vi "Nonlinear Calibration Test v4.vi"() -> ()   [LabVIEW 2009]
doc: "This example illustrates the use of a calibration grid to calibrate and correct an image for nonlinear distortion and accurate shape measurements.\n\nThis example loads the image of a calibration grid used to calibrate the system, learns the grid, then loads an image of parts acquired using the same setup. The example then corrects the image in two ways. The first method corrects the entire image and then measures the area of the coins. The second method corrects only the area of the coins and displays the difference in processing time."
uses:
  <vilib>/userDefined/High Color/IMAQdx.ctl
  <vilib>/vision/NI_Vision_Development_Module.lvlib
  <vilib>/vision/driver/NI_Vision_Acquisition_Software.lvlib
panel:
  in  "Camera Name":T1
  in  "Video Modes":i32(listbox)
  in  "stop":bool
  out "Image":T2(plugin-control)
  out "Buffer Number":u32
  out "Frame Rate":dbl(knob) scale=0.0..100.0 scale format="%.1f"
  in  "Red Range":cluster{"Lower value":i32, "Upper value":i32}={"Lower value"=240, "Upper value"=255}
  in  "Green Range":cluster{"Lower value":i32, "Upper value":i32}={"Lower value"=250, "Upper value"=255}
  in  "Blue Range":cluster{"Lower value":i32, "Upper value":i32}={"Lower value"=250, "Upper value"=255}
  in  "Color Mode":u16(ring) items=["RGB", "HSL", "HSV", "HSI"]
  out "Super Filter":T2(plugin-control)
  in  "File Path 2":path
  in  "File Path":path
  out "Bottom Image":T2(plugin-control) caption="Calibrated Measurements"
  out "Top Image":T2(plugin-control) caption="Corrected Image"
  # "This step takes measurements in two ways.  The first calculation corrects \nthe entire image, and then takes the measurements.  The second calculation only corrects the coins, and then takes the measurements."
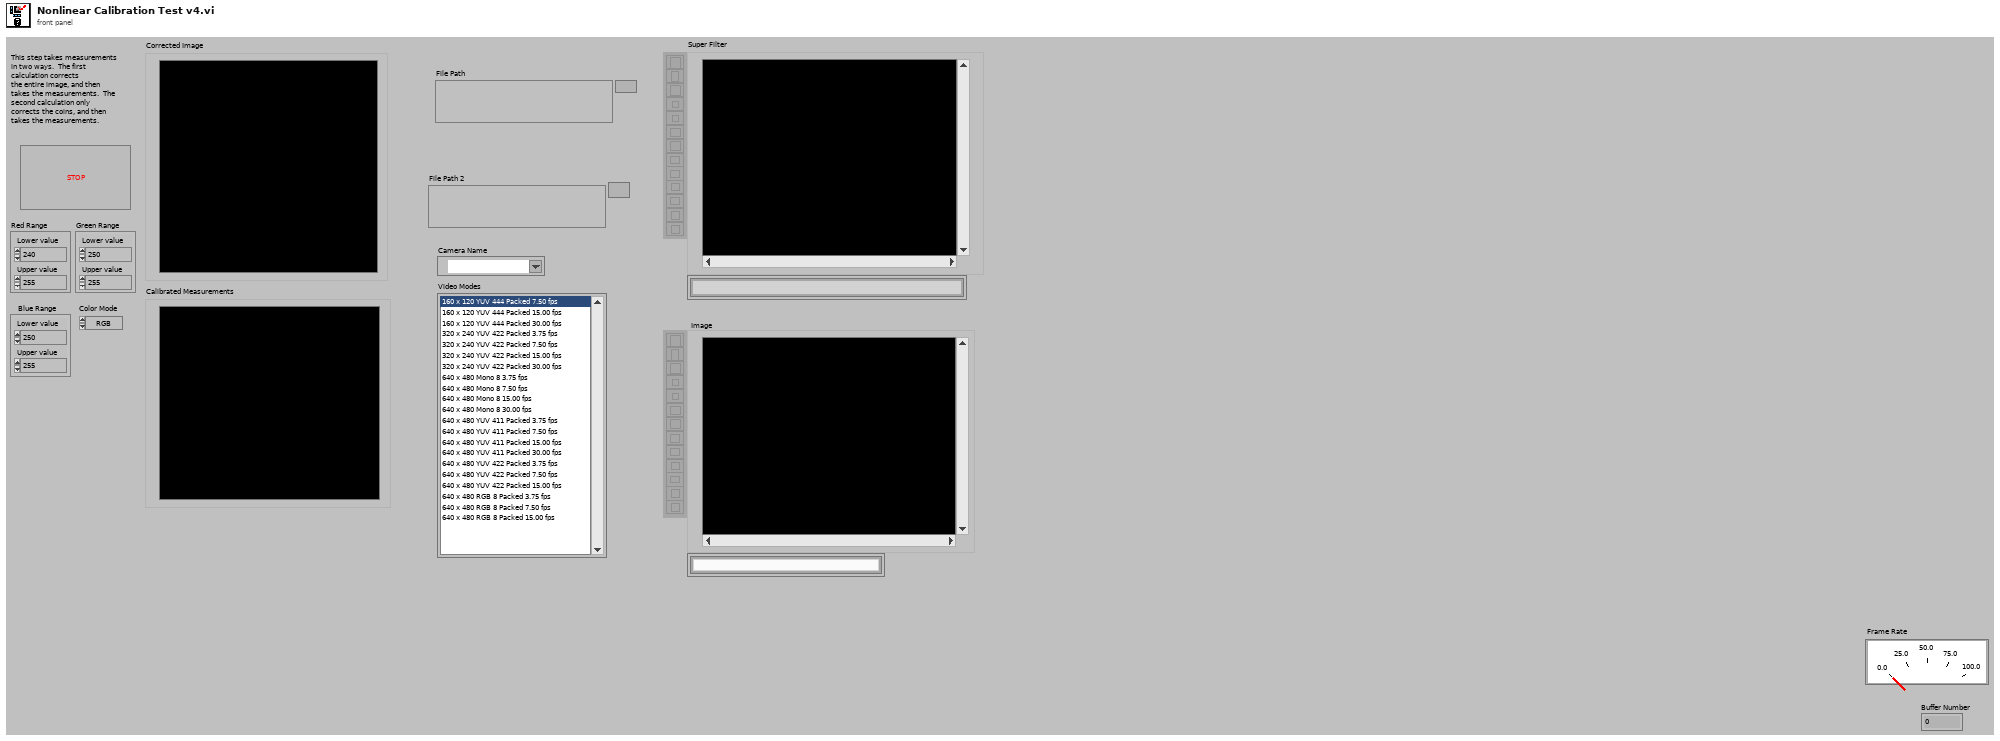
[diagram p1: front panel]
types:
  T1 = typedef "IMAQdx.ctl" = refnum<k21>
  T2 = typedef "IMAQ Image.ctl" = refnum<image>
  T3 = typedef "Image Type" = u32
  T4 = cluster{"X Step":sgl, "Y Step":sgl, "Unit":u32, "Threshold Range":cluster{"Lower value":sgl, "Upper value":sgl}}
  T5 = cluster{"Distortion":u32, "Corrected Image Scaling":u32, "Corrected Image Learn ROI":u32, "Learn Error Map?":bool, "Learn Correction Table?":bool}
  T6 = typedef "Particle Parameters" = i32
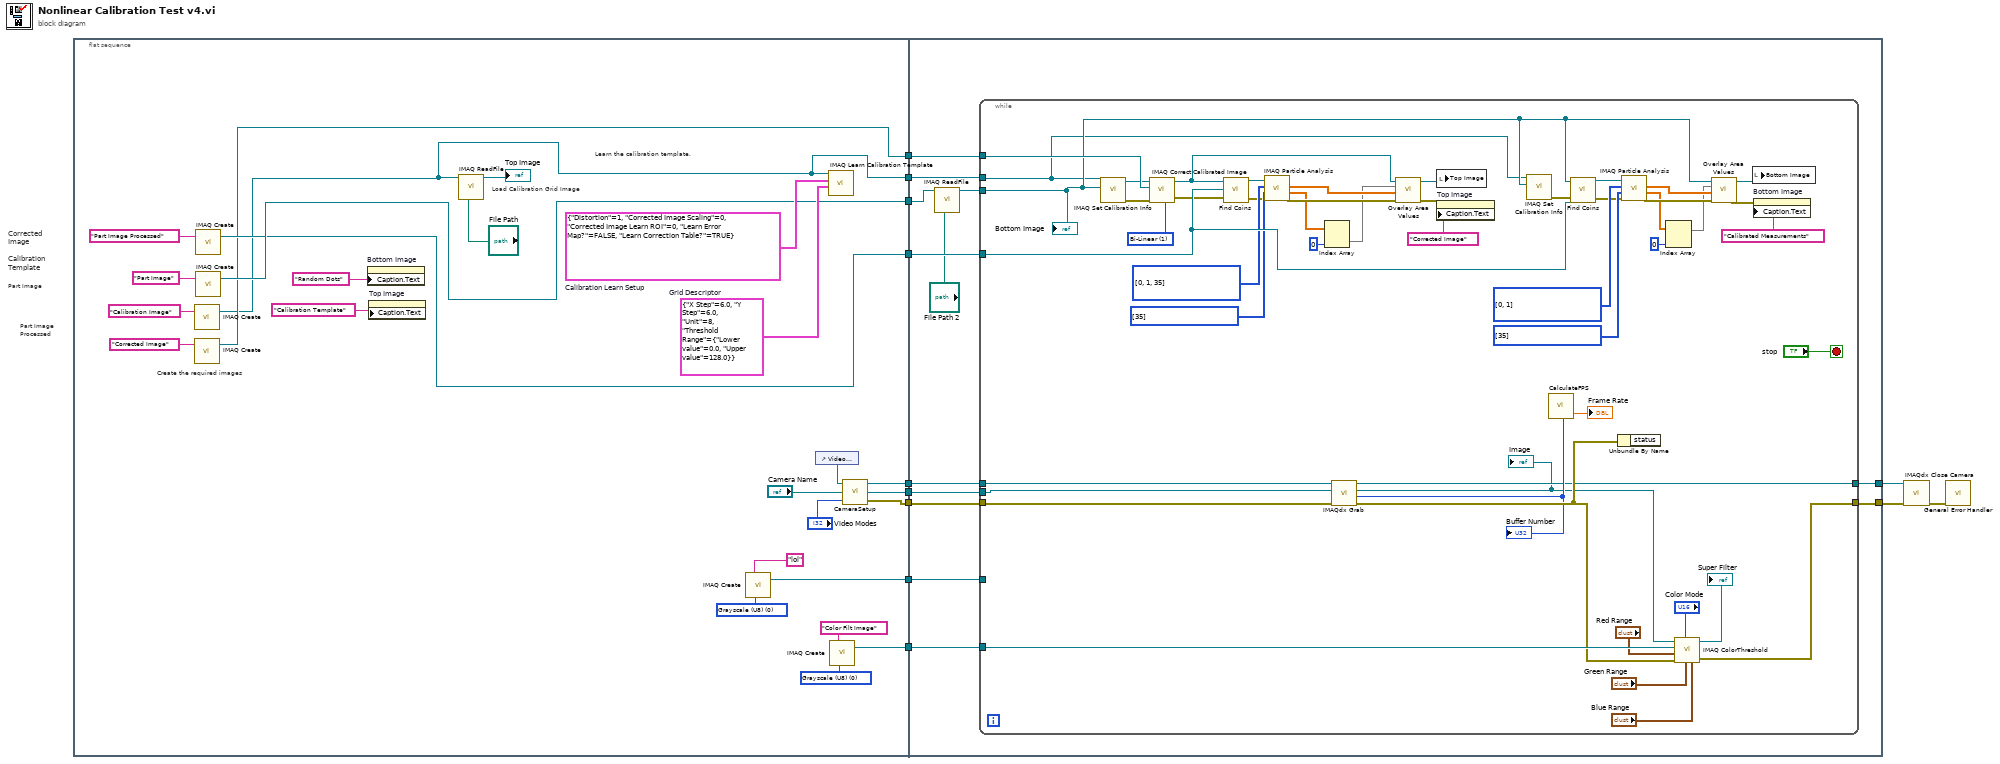
[diagram p0: block diagram]
diagram:
  # "Corrected\nImage"
  # "Part Image Processed"
  # "Calibration Template"
  # "Part Image"
  n1 = flat-sequence {
    tunnel: [w36] -> w12
    tunnel: [w21] -> w11
    tunnel: [w35] -> w10
    tunnel: [w26] -> w9
    tunnel: [w22] -> w5
    tunnel: [w19] -> w4
    tunnel: [w18] -> w3
    tunnel: [w17] -> w2
    tunnel: [w13] -> w1
    tunnel: w12 -> [w47]
    tunnel: w11 -> [w51]
    tunnel: w10 -> [w50]
    tunnel: w9 -> [w49]
    tunnel: [w45] -> w7
    tunnel: [w44] -> w6
    tunnel: w5 -> [w43]
    tunnel: w4 -> [w42]
    tunnel: w3 -> [w41]
    tunnel: w2 -> [w40]
    tunnel: w1 -> [w39]
    frame #0 {
      w15 = T3 0 items=["Grayscale (U8)", "Grayscale (I16)", "Grayscale (SGL)", "Complex (CSG)", "RGB (U32)", "HSL (U32)", "RGB (U64)", "Grayscale (U16)"] ("Image Type")
      w25 = T3 0 items=["Grayscale (U8)", "Grayscale (I16)", "Grayscale (SGL)", "Complex (CSG)", "RGB (U32)", "HSL (U32)", "RGB (U64)", "Grayscale (U16)"] ("Image Type")
      w37 = T4 {"X Step"=6.0, "Y Step"=6.0, "Unit"=8, "Threshold Range"={"Lower value"=0.0, "Upper value"=128.0}}  # Grid Descriptor
      w38 = T5 {"Distortion"=1, "Corrected Image Scaling"=0, "Corrected Image Learn ROI"=0, "Learn Error Map?"=FALSE, "Learn Correction Table?"=TRUE}  # Calibration Learn Setup
      # "Create the required images"
      # "Load Calibration Grid Image"
      # "Learn the calibration template."
      n2 = call "IMAQ Create"("Image Name"="Calibration Image") -> ("New Image"=w21:T2)  [unwired: 3 in, 2 out]
      n3 = call "IMAQ Create"("Image Name"="Corrected Image") -> ("New Image"=w26:T2)  [unwired: 3 in, 2 out]
      n4 = call "IMAQ Create"("Image Name"="Part Image Processed") -> ("New Image"=w35:T2)  [unwired: 3 in, 2 out]
      n5 = call "IMAQ Create"("Image Name"="Part Image") -> ("New Image"=w36:T2)  [unwired: 3 in, 2 out]
      n6 = property on="Bottom Image" class="ImageControl"("Caption.Text"="Random Dots" ("Title")) -> ()  [unwired: 2 in, 2 out]
      n7 = property on="Top Image" class="ImageControl"("Caption.Text"="Calibration Template" ("Title")) -> ()  [unwired: 2 in, 2 out]
      n8 = call "IMAQ ReadFile"("File Path"="File Path", "Image"=w21) -> ("Image Out"=→"Top Image":T2)  [unwired: 3 in, 6 out]
      n9 = call "IMAQ Create"("Image Name"="lol", "Image Type"=w15) -> ("New Image"=w13:T2)  [unwired: 2 in, 2 out]
      n10 = control-ref of="Video Modes"() -> (w16:refnum<vi>)
      n11 = call "IMAQ Learn Calibration Template"("Grid Descriptor"=w37, "Calibration Learn Setup"=w38, "Image"=w21) -> ()  [unwired: 4 in, 5 out]
      n12 = call "IMAQ Create"("Image Name"="Color Filt Image", "Image Type"=w25) -> ("New Image"=w22:T2)  [unwired: 2 in, 2 out]
      n13 = call "CameraSetup.vi"("Video Modes"="Video Modes", "Camera Name"="Camera Name", "reference"=w16) -> ("error out"=w17:errorcluster, "New Image"=w18:T2, "Session Out"=w19:T1)
    }
    frame #1 {
      n14 = call "IMAQ ReadFile"("File Path"="File Path 2", "Image"=w47) -> ("Image Out"=w46:T2)  [unwired: 3 in, 6 out]
      n15 = while {
        tunnel: w51 -> [w52]
        tunnel: w50 -> [w101]
        tunnel: w49 -> [w89]
        tunnel: w43 -> [w77]
        tunnel: w46 -> [w76]
        tunnel: [w57] -> w45
        tunnel: [w61] -> w44
        tunnel: w42 -> [w56]
        tunnel: w41 -> [w55]
        tunnel: w40 -> [w54]
        tunnel: w39 -> [_]
        stop <- "stop" stop-if-true
        w81 = u32 1 items=["Zero Order", "Bi-Linear", "Quadratic", "Cubic Spline"] ("Interpolation Type")
        w88 = T6[] [0, 1, 35] items=["Center of Mass X", "Center of Mass Y", "First Pixel X", "First Pixel Y", "Bounding Rect Left", "Bounding Rect Top", "Bounding Rect Right", "Bounding Rect Bottom", "Max Feret Diameter Start X", "Max Feret Diameter Start Y", "Max Feret Diameter End X", "Max Feret Diameter End Y", "Max Horiz. Segment Length Left", "Max Horiz. Segment Length Right", "Max Horiz. Segment Length Row", "-", "Bounding Rect Width", "Bounding Rect Height", "Bounding Rect Diagonal", "Perimeter", "Convex Hull Perimeter", "Holes' Perimeter", "Max Feret Diameter", "Equivalent Ellipse Major Axis", "Equivalent Ellipse Minor Axis", "Equivalent Ellipse Minor Axis (Feret)", "Equivalent Rect Long Side", "Equivalent Rect Short Side", "Equivalent Rect Diagonal", "Equivalent Rect Short Side (Feret)", "Average Horiz. Segment Length", "Average Vert. Segment Length", "Hydraulic Radius", "Waddel Disk Diameter", "-", "Area", "Holes' Area", "Particle & Holes' Area", "Convex Hull Area", "Image Area", "-", "Number of Holes", "Number of Horiz. Segments", "Number of Vert. Segments", "-", "Orientation", "Max Feret Diameter Orientation", "-", "% Area/Image Area", "% Area/(Particle & Holes' Area)", "Ratio of Equivalent Ellipse Axes", "Ratio of Equivalent Rect Sides", "-", "Elongation Factor", "Compactness Factor", "Heywood Circularity Factor", "Type Factor", "-", "Sum X", "Sum Y", "Sum XX", "Sum XY", "Sum YY", "Sum XXX", "Sum XXY", "Sum XYY", "Sum YYY", "-", "Moment of Inertia XX", "Moment of Inertia XY", "Moment of Inertia YY", "Moment of Inertia XXX", "Moment of Inertia XXY", "Moment of Inertia XYY", "Moment of Inertia YYY", "Norm. Moment of Inertia XX", "Norm. Moment of Inertia XY", "Norm. Moment of Inertia YY", "Norm. Moment of Inertia XXX", "Norm. Moment of Inertia XXY", "Norm. Moment of Inertia XYY", "Norm. Moment of Inertia YYY", "Hu Moment 1", "Hu Moment 2", "Hu Moment 3", "Hu Moment 4", "Hu Moment 5", "Hu Moment 6", "Hu Moment 7"] ("Calibrated Measurements")
        w87 = T6[] [35] items=["Center of Mass X", "Center of Mass Y", "First Pixel X", "First Pixel Y", "Bounding Rect Left", "Bounding Rect Top", "Bounding Rect Right", "Bounding Rect Bottom", "Max Feret Diameter Start X", "Max Feret Diameter Start Y", "Max Feret Diameter End X", "Max Feret Diameter End Y", "Max Horiz. Segment Length Left", "Max Horiz. Segment Length Right", "Max Horiz. Segment Length Row", "-", "Bounding Rect Width", "Bounding Rect Height", "Bounding Rect Diagonal", "Perimeter", "Convex Hull Perimeter", "Holes' Perimeter", "Max Feret Diameter", "Equivalent Ellipse Major Axis", "Equivalent Ellipse Minor Axis", "Equivalent Ellipse Minor Axis (Feret)", "Equivalent Rect Long Side", "Equivalent Rect Short Side", "Equivalent Rect Diagonal", "Equivalent Rect Short Side (Feret)", "Average Horiz. Segment Length", "Average Vert. Segment Length", "Hydraulic Radius", "Waddel Disk Diameter", "-", "Area", "Holes' Area", "Particle & Holes' Area", "Convex Hull Area", "Image Area", "-", "Number of Holes", "Number of Horiz. Segments", "Number of Vert. Segments", "-", "Orientation", "Max Feret Diameter Orientation", "-", "% Area/Image Area", "% Area/(Particle & Holes' Area)", "Ratio of Equivalent Ellipse Axes", "Ratio of Equivalent Rect Sides", "-", "Elongation Factor", "Compactness Factor", "Heywood Circularity Factor", "Type Factor", "-", "Sum X", "Sum Y", "Sum XX", "Sum XY", "Sum YY", "Sum XXX", "Sum XXY", "Sum XYY", "Sum YYY", "-", "Moment of Inertia XX", "Moment of Inertia XY", "Moment of Inertia YY", "Moment of Inertia XXX", "Moment of Inertia XXY", "Moment of Inertia XYY", "Moment of Inertia YYY", "Norm. Moment of Inertia XX", "Norm. Moment of Inertia XY", "Norm. Moment of Inertia YY", "Norm. Moment of Inertia XXX", "Norm. Moment of Inertia XXY", "Norm. Moment of Inertia XYY", "Norm. Moment of Inertia YYY", "Hu Moment 1", "Hu Moment 2", "Hu Moment 3", "Hu Moment 4", "Hu Moment 5", "Hu Moment 6", "Hu Moment 7"] ("Pixel Measurements")
        w95 = T6[] [0, 1] items=["Center of Mass X", "Center of Mass Y", "First Pixel X", "First Pixel Y", "Bounding Rect Left", "Bounding Rect Top", "Bounding Rect Right", "Bounding Rect Bottom", "Max Feret Diameter Start X", "Max Feret Diameter Start Y", "Max Feret Diameter End X", "Max Feret Diameter End Y", "Max Horiz. Segment Length Left", "Max Horiz. Segment Length Right", "Max Horiz. Segment Length Row", "-", "Bounding Rect Width", "Bounding Rect Height", "Bounding Rect Diagonal", "Perimeter", "Convex Hull Perimeter", "Holes' Perimeter", "Max Feret Diameter", "Equivalent Ellipse Major Axis", "Equivalent Ellipse Minor Axis", "Equivalent Ellipse Minor Axis (Feret)", "Equivalent Rect Long Side", "Equivalent Rect Short Side", "Equivalent Rect Diagonal", "Equivalent Rect Short Side (Feret)", "Average Horiz. Segment Length", "Average Vert. Segment Length", "Hydraulic Radius", "Waddel Disk Diameter", "-", "Area", "Holes' Area", "Particle & Holes' Area", "Convex Hull Area", "Image Area", "-", "Number of Holes", "Number of Horiz. Segments", "Number of Vert. Segments", "-", "Orientation", "Max Feret Diameter Orientation", "-", "% Area/Image Area", "% Area/(Particle & Holes' Area)", "Ratio of Equivalent Ellipse Axes", "Ratio of Equivalent Rect Sides", "-", "Elongation Factor", "Compactness Factor", "Heywood Circularity Factor", "Type Factor", "-", "Sum X", "Sum Y", "Sum XX", "Sum XY", "Sum YY", "Sum XXX", "Sum XXY", "Sum XYY", "Sum YYY", "-", "Moment of Inertia XX", "Moment of Inertia XY", "Moment of Inertia YY", "Moment of Inertia XXX", "Moment of Inertia XXY", "Moment of Inertia XYY", "Moment of Inertia YYY", "Norm. Moment of Inertia XX", "Norm. Moment of Inertia XY", "Norm. Moment of Inertia YY", "Norm. Moment of Inertia XXX", "Norm. Moment of Inertia XXY", "Norm. Moment of Inertia XYY", "Norm. Moment of Inertia YYY", "Hu Moment 1", "Hu Moment 2", "Hu Moment 3", "Hu Moment 4", "Hu Moment 5", "Hu Moment 6", "Hu Moment 7"] ("Calibrated Measurements")
        w99 = T6[] [35] items=["Center of Mass X", "Center of Mass Y", "First Pixel X", "First Pixel Y", "Bounding Rect Left", "Bounding Rect Top", "Bounding Rect Right", "Bounding Rect Bottom", "Max Feret Diameter Start X", "Max Feret Diameter Start Y", "Max Feret Diameter End X", "Max Feret Diameter End Y", "Max Horiz. Segment Length Left", "Max Horiz. Segment Length Right", "Max Horiz. Segment Length Row", "-", "Bounding Rect Width", "Bounding Rect Height", "Bounding Rect Diagonal", "Perimeter", "Convex Hull Perimeter", "Holes' Perimeter", "Max Feret Diameter", "Equivalent Ellipse Major Axis", "Equivalent Ellipse Minor Axis", "Equivalent Ellipse Minor Axis (Feret)", "Equivalent Rect Long Side", "Equivalent Rect Short Side", "Equivalent Rect Diagonal", "Equivalent Rect Short Side (Feret)", "Average Horiz. Segment Length", "Average Vert. Segment Length", "Hydraulic Radius", "Waddel Disk Diameter", "-", "Area", "Holes' Area", "Particle & Holes' Area", "Convex Hull Area", "Image Area", "-", "Number of Holes", "Number of Horiz. Segments", "Number of Vert. Segments", "-", "Orientation", "Max Feret Diameter Orientation", "-", "% Area/Image Area", "% Area/(Particle & Holes' Area)", "Ratio of Equivalent Ellipse Axes", "Ratio of Equivalent Rect Sides", "-", "Elongation Factor", "Compactness Factor", "Heywood Circularity Factor", "Type Factor", "-", "Sum X", "Sum Y", "Sum XX", "Sum XY", "Sum YY", "Sum XXX", "Sum XXY", "Sum XYY", "Sum YYY", "-", "Moment of Inertia XX", "Moment of Inertia XY", "Moment of Inertia YY", "Moment of Inertia XXX", "Moment of Inertia XXY", "Moment of Inertia XYY", "Moment of Inertia YYY", "Norm. Moment of Inertia XX", "Norm. Moment of Inertia XY", "Norm. Moment of Inertia YY", "Norm. Moment of Inertia XXX", "Norm. Moment of Inertia XXY", "Norm. Moment of Inertia XYY", "Norm. Moment of Inertia YYY", "Hu Moment 1", "Hu Moment 2", "Hu Moment 3", "Hu Moment 4", "Hu Moment 5", "Hu Moment 6", "Hu Moment 7"] ("Pixel Measurements")
        n16 = call "IMAQ Set Calibration Info"("Image Dst"=w76, "Image Src"=w52) -> ("error out"=w74:errorcluster, "Calibrated Image"=w75:T2)  [unwired: 2 in, 6 out]
        n17 = call "IMAQ Correct Calibrated Image"("Interpolation Type"=w81, "error in (no error)"=w74, "Image Dst"=w89, "Image Src"=w75) -> ("error out"=w73:errorcluster, "Corrected Image"=w82:T2)  [unwired: 3 in, 3 out]
        n18 = call "Find Coins.vi"("error in"=w73, "Dest Image"=w101, "Source Image"=w82) -> ("error out"=w72:errorcluster, "Image Out"=w71:T2)  [unwired: 1 out]
        n19 = call "IMAQ Particle Analysis"("error in (no error)"=w72, "Real-World Measurements"=w87, "Pixel Measurements"=w88, "Image"=w71) -> ("error out"=w90:errorcluster, "Particle Measurements (Real-World)"=w84:dbl[][], "Particle Measurements (Pixels)"=w86:dbl[][])  [unwired: 1 in, 4 out]
        n20 = Index Array(array=w84, index (col)=0 ("Index (row)")) -> (element=w85:dbl[])  [unwired: 1 in]
        n21 = call <vilib>:"IMAQdx Grab.vi"("error in"=w54, "Image In"=w55, "Session In"=w56) -> ("error out"=w59:errorcluster, "Buffer Number Out"=w58:u32, "Image Out"=w53:T2, "Session Out"=w57:T1)  [unwired: 1 in, 4 out]
        "Image" <- w53
        "Buffer Number" <- w58
        n22 = call "Overlay Area Values.vi"("error in (no error)"=w90, "Coin Center (X,Y)"=w86, "Measurement Values"=w85, "Image In"=w82) -> ("error out"=w79:errorcluster, "Image Out"=w80:T2)  [unwired: 2 out]
        n23 = local write "Top Image"(w80) -> ()
        n24 = property on="Top Image" class="ImageControl"(error in=w79, "Caption.Text"="Corrected Image" ("Title")) -> ()  [unwired: 1 in, 2 out]
        n25 = call "IMAQ Set Calibration Info"("Image Dst"=w76, "Image Src"=w52) -> ("error out"=w68:errorcluster)  [unwired: 2 in, 7 out]
        n26 = call "CalculateFPS.vi"("buffer number"=w58) -> ("processed FPS"=→"Frame Rate":dbl)  [unwired: 2 out]
        n27 = call "Find Coins.vi"("error in"=w68, "Dest Image"=w101, "Source Image"=w76) -> ("error out"=w70:errorcluster, "Image Out"=w69:T2)  [unwired: 1 out]
        n28 = Unbundle By Name(w59) -> ()  [unwired: 1 out]
        n29 = call "IMAQ Particle Analysis"("error in (no error)"=w70, "Real-World Measurements"=w99, "Pixel Measurements"=w95, "Image"=w69) -> ("error out"=w100:errorcluster, "Particle Measurements (Real-World)"=w97:dbl[][], "Particle Measurements (Pixels)"=w98:dbl[][])  [unwired: 1 in, 4 out]
        n30 = Index Array(array=w97, index (col)=0 ("Index (row)")) -> (element=w94:dbl[])  [unwired: 1 in]
        n31 = call "IMAQ ColorThreshold"("Blue or Luma or Val or Inten Range"="Blue Range", "Green or Sat Range"="Green Range", "Color Mode"="Color Mode", "error in (no error)"=w59, "Red or Hue Range"="Red Range", "Image Dst"=w77, "Image Src"=w53) -> ("error out"=w61:errorcluster, "Image Dst Out"=→"Super Filter":T2)  [unwired: 3 in]
        n32 = call "Overlay Area Values.vi"("error in (no error)"=w100, "Coin Center (X,Y)"=w98, "Measurement Values"=w94, "Image In"=w76) -> ("error out"=w92:errorcluster, "Image Out"=w93:T2)  [unwired: 2 out]
        n33 = local write "Bottom Image"(w93) -> ()
        n34 = property on="Bottom Image" class="ImageControl"(error in=w92, "Caption.Text"="Calibrated Measurements" ("Title")) -> ()  [unwired: 1 in, 2 out]
        "Bottom Image" <- w76
      }
    }
  }
  n35 = call <vilib>:"IMAQdx Close Camera.vi"("error in"=w6, "Session In"=w7) -> ("error out"=w8:errorcluster)  [unwired: 9 out]
  n36 = call <vilib>:"General Error Handler.vi"("error in (no error)"=w8) -> ()  [unwired: 1 in, 14 out]
